vi "RT_Configuration(FGV).vi"(6 "File Method":T2, 8 "error in":errorcluster, 11 "Configuration In":T1) -> (0 "error out":errorcluster, 3 "Configuration Out":T1)   [LabVIEW 2018]
uses:
  Data Def/RT_File Method.ctl
  Data Def/RT_Configuration.ctl
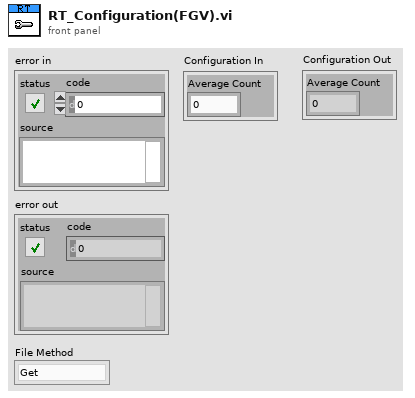
[diagram p1: front panel]
types:
  T1 = typedef "RT_Configuration.ctl" = cluster{"Average Count":i32}
  T2 = typedef "RT_File Method.ctl" = enum16{"Get", "Put", "Load", "Save"}
  T3 = enum16{"open", "replace", "create", "open or create", "replace or create", "replace or create with confirmation"}
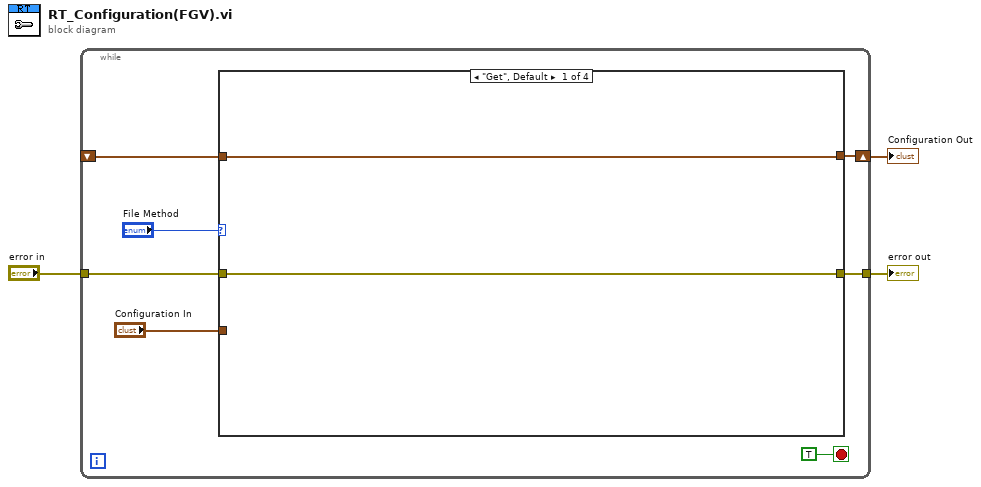
[diagram p0: block diagram]
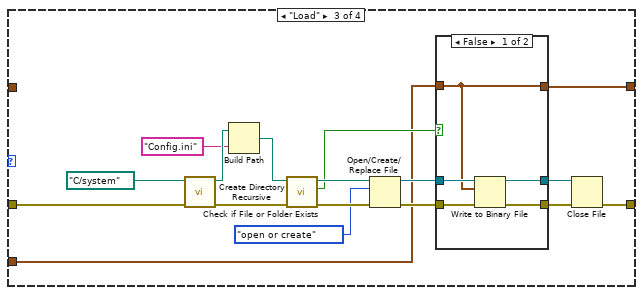
[diagram p3: hidden frame]
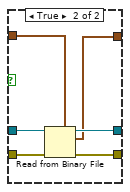
[diagram p4: hidden frame]
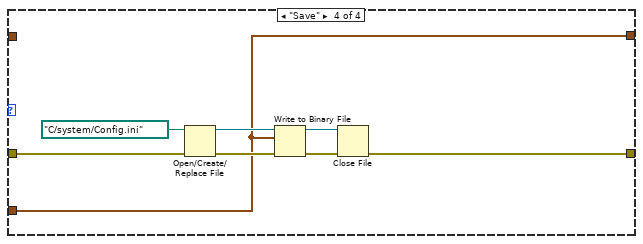
[diagram p5: hidden frame]
diagram:
  n1 = while {
    tunnel: "error in" -> [w8]
    shift-right: [w6] -> w2
    shift-left: _ -> [w4]
    tunnel: [w5] -> w1
    stop <- TRUE stop-if-true
    n2 = case shown="\"Get\", Default" "File Method" {
      tunnel: w8 -> [w11 w14 w28 w50]
      tunnel: "Configuration In" -> [_ w13 w19 w46]
      tunnel: [w12 w13 w18 w46] -> w6
      tunnel: [w11 w14 w15 w43] -> w5
      tunnel: w4 -> [w12 _ _ _]
      frame "Get", Default {
      }
      frame "Put" {
      }
      frame "Load" {
        n3 = call <vilib>:"Create Directory Recursive.vi"("error in (no error)"=w28, "directory"=path "C:/system") -> ("error out"=w27:errorcluster, "directory copy"=w31:path)  [unwired: 3 in, 1 out]
        n4 = Build Path(base path=w31, name or relative path="Config.ini") -> (appended path=w26:path)
        n5 = call <vilib>:"Check if File or Folder Exists.vi"("error in (no error)"=w27, "path"=w26) -> ("error out"=w25:errorcluster, "file or folder exists?"=w22:bool, "dup path"=w24:path)  [unwired: 7 in]
        n6 = Open/Create/Replace File(file path (use dialog)=w24, error in=w25, operation (0:open)=T3."open or create") -> (refnum out=w21:refnum<file>, error out=w20:errorcluster)  [unwired: 3 in, 1 out]
        n7 = case shown="False" w22 {
          tunnel: w21 -> [w35 w41]
          tunnel: w20 -> [w36 w42]
          tunnel: w19 -> [w32 w38]
          tunnel: [w34 w39] -> w16
          tunnel: [w33 w40] -> w17
          tunnel: [w32 w37] -> w18
          frame False {
            n8 = Write to Binary File(file (use dialog)=w35, data=w32, error in=w36) -> (refnum out=w34:refnum<file>, error out=w33:errorcluster)  [unwired: 3 in, 1 out]
          }
          frame True {
            n9 = Read from Binary File(5:w38, 8:w42, 11:w41) -> (0:w40:errorcluster, 2:w37:T1, 3:w39:refnum<file>)  [unwired: 3 in, 1 out]
          }
        }
        n10 = Close File(refnum=w16, error in=w17) -> (error out=w15:errorcluster)  [unwired: 1 out]
      }
      frame "Save" {
        n11 = Open/Create/Replace File(file path (use dialog)=path "C:/system/Config.ini", error in=w50) -> (refnum out=w47:refnum<file>, error out=w48:errorcluster)  [unwired: 4 in, 1 out]
        n12 = Write to Binary File(file (use dialog)=w47, data=w46, error in=w48) -> (refnum out=w44:refnum<file>, error out=w45:errorcluster)  [unwired: 3 in, 1 out]
        n13 = Close File(refnum=w44, error in=w45) -> (error out=w43:errorcluster)  [unwired: 1 out]
      }
    }
  }
  "error out" <- w1
  "Configuration Out" <- w2
